vi "HIS_to_DAT_to_TRABS.vi"() -> ()   [LabVIEW 2015]
uses:
  DATA/HIS/HIS.lvclass
  dependecies/HIS_to_DAT_to_TRABS/cluster_template.ctl
panel:
  in  "file name TRABS":string
  in  "file name modifier DAT":string
  out "CERENKOV_unsel":T1(graph)
  out "BRUIT_unsel":T1(graph)
  out "BASE_sel":T1(graph)
  out "ABS_unsel":T1(graph)
  in  "select":bool caption="Lock"
  in  "Save TRABS":bool
  in  "Play":bool
  in  "Fast Forward":bool
  in  "Fast Reverse":bool
  in  "Skip to End":bool
  in  "Skip to Beginning":bool
  out "#CERENKOV":i32
  out "#BRUIT":i32
  out "#BASE":i32
  out "#ABS":i32
  in  "MAIN_path":path
  out "error out":errorcluster
  in  "to TRABS":bool
  out "TRABS":dbl[][](graph)
  in  "CERENKOV_b":bool
  in  "BRUIT_b":bool
  in  "BASE_b":bool
  out "CERENKOV_path":path
  out "BRUIT_path":path
  in  "stop_vi":bool
  in  "ABS_b":bool
  in  "All":bool
  in  "deselect":bool=TRUE caption="Lock"
  in  "Save DAT":bool
  out "BASE_path":path
  out "ABS_path":path
  out "CERENKOV DAT":dbl[][](graph)
  out "BRUIT DAT":dbl[][](graph)
  out "BASE DAT":dbl[][](graph)
  out "ABS DAT":dbl[][](graph)
  out "CERENKOV HIS":dbl[][](graph)
  out "BRUIT HIS":dbl[][](graph)
  out "BASE HIS":dbl[][](graph)
  in  "to Dat":bool
  out "ABS HIS":dbl[][](graph)
  out "Slide":u8(slide) scale=0.0..100.0
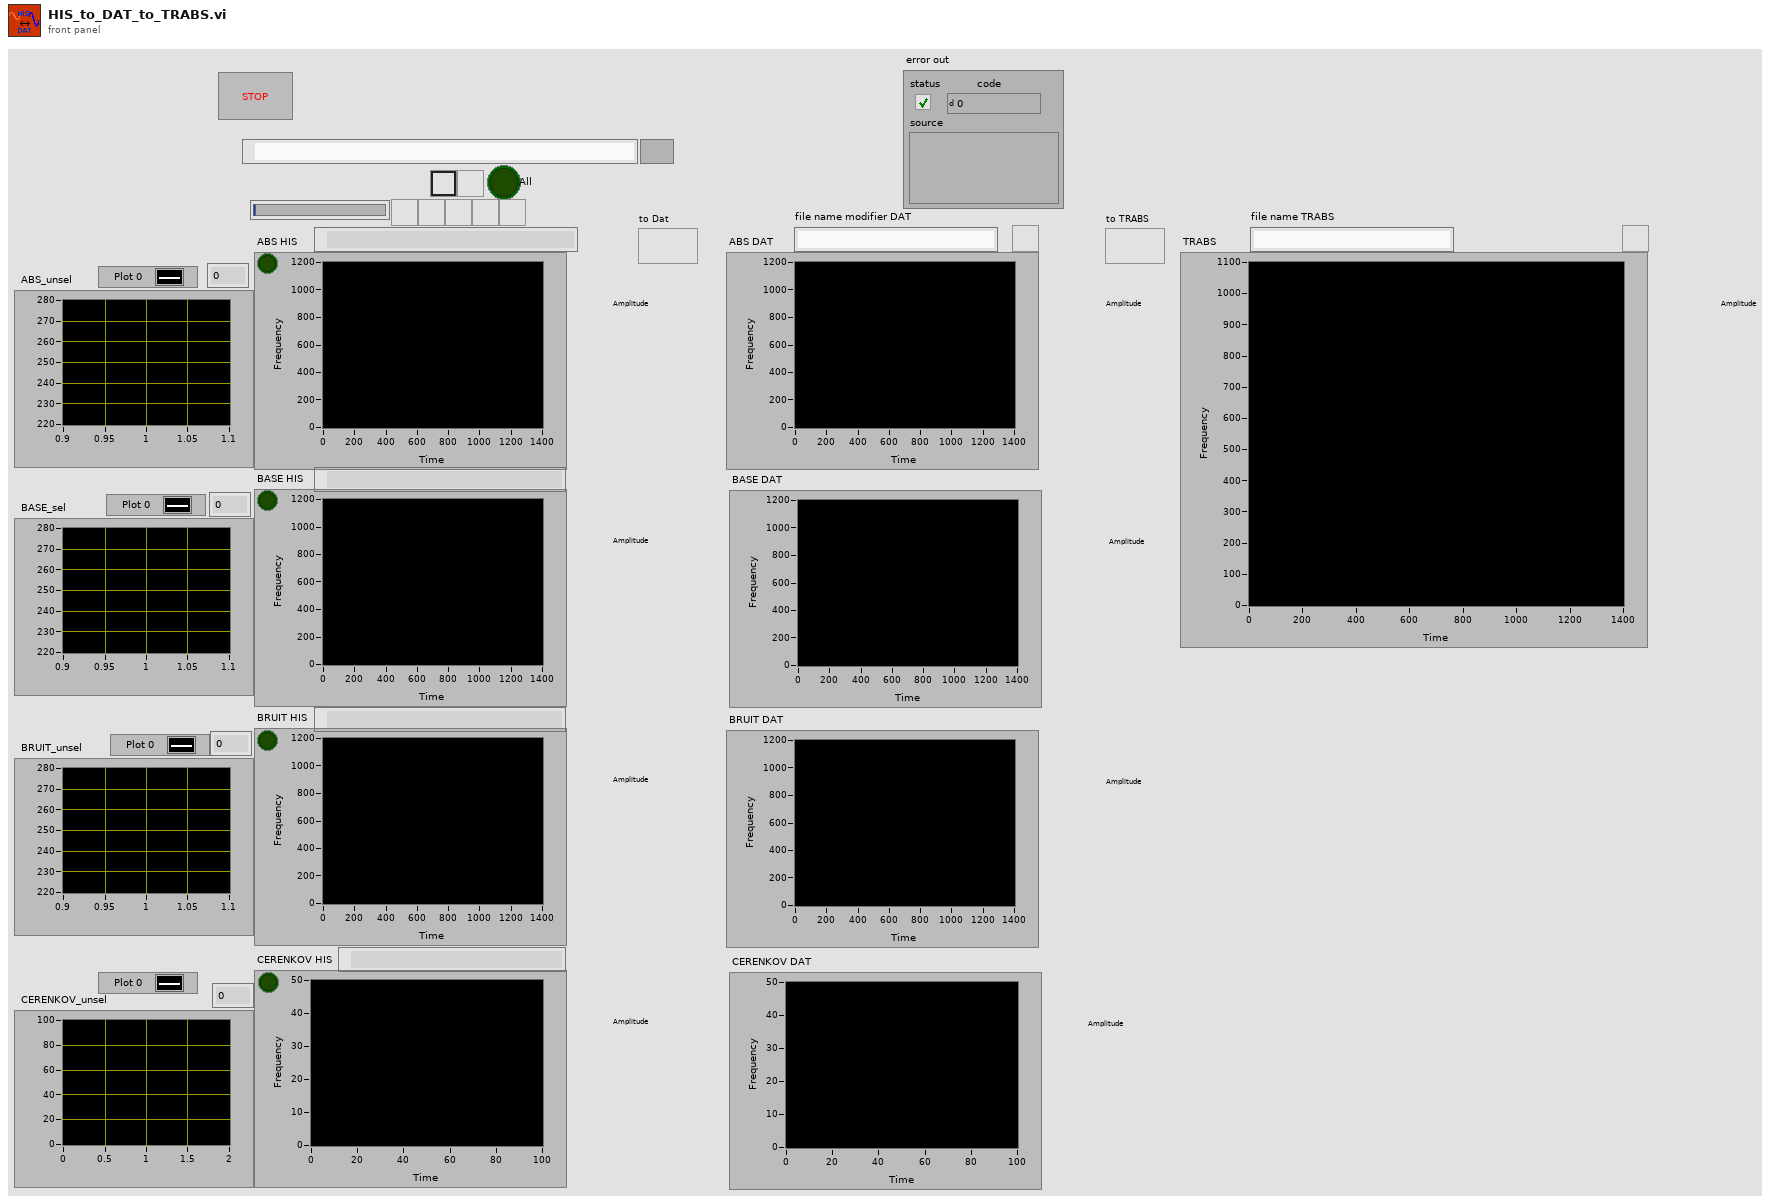
[diagram p1: front panel]
types:
  T1 = cluster{"appended array":dbl[], "appended array":dbl[]}
  T2 = typedef "cluster_template.ctl" = cluster{"HIS.lvclass":refnum<class "HIS.lvclass">, "selector":refnum<vi>, "HIS graph":refnum<vi>, "DAT graph":refnum<vi>, "path":refnum<vi>, "path MAIN":refnum<vi>, "#":refnum<vi>, "unsel Graph":refnum<vi>, "DATgraph":refnum<vi>}
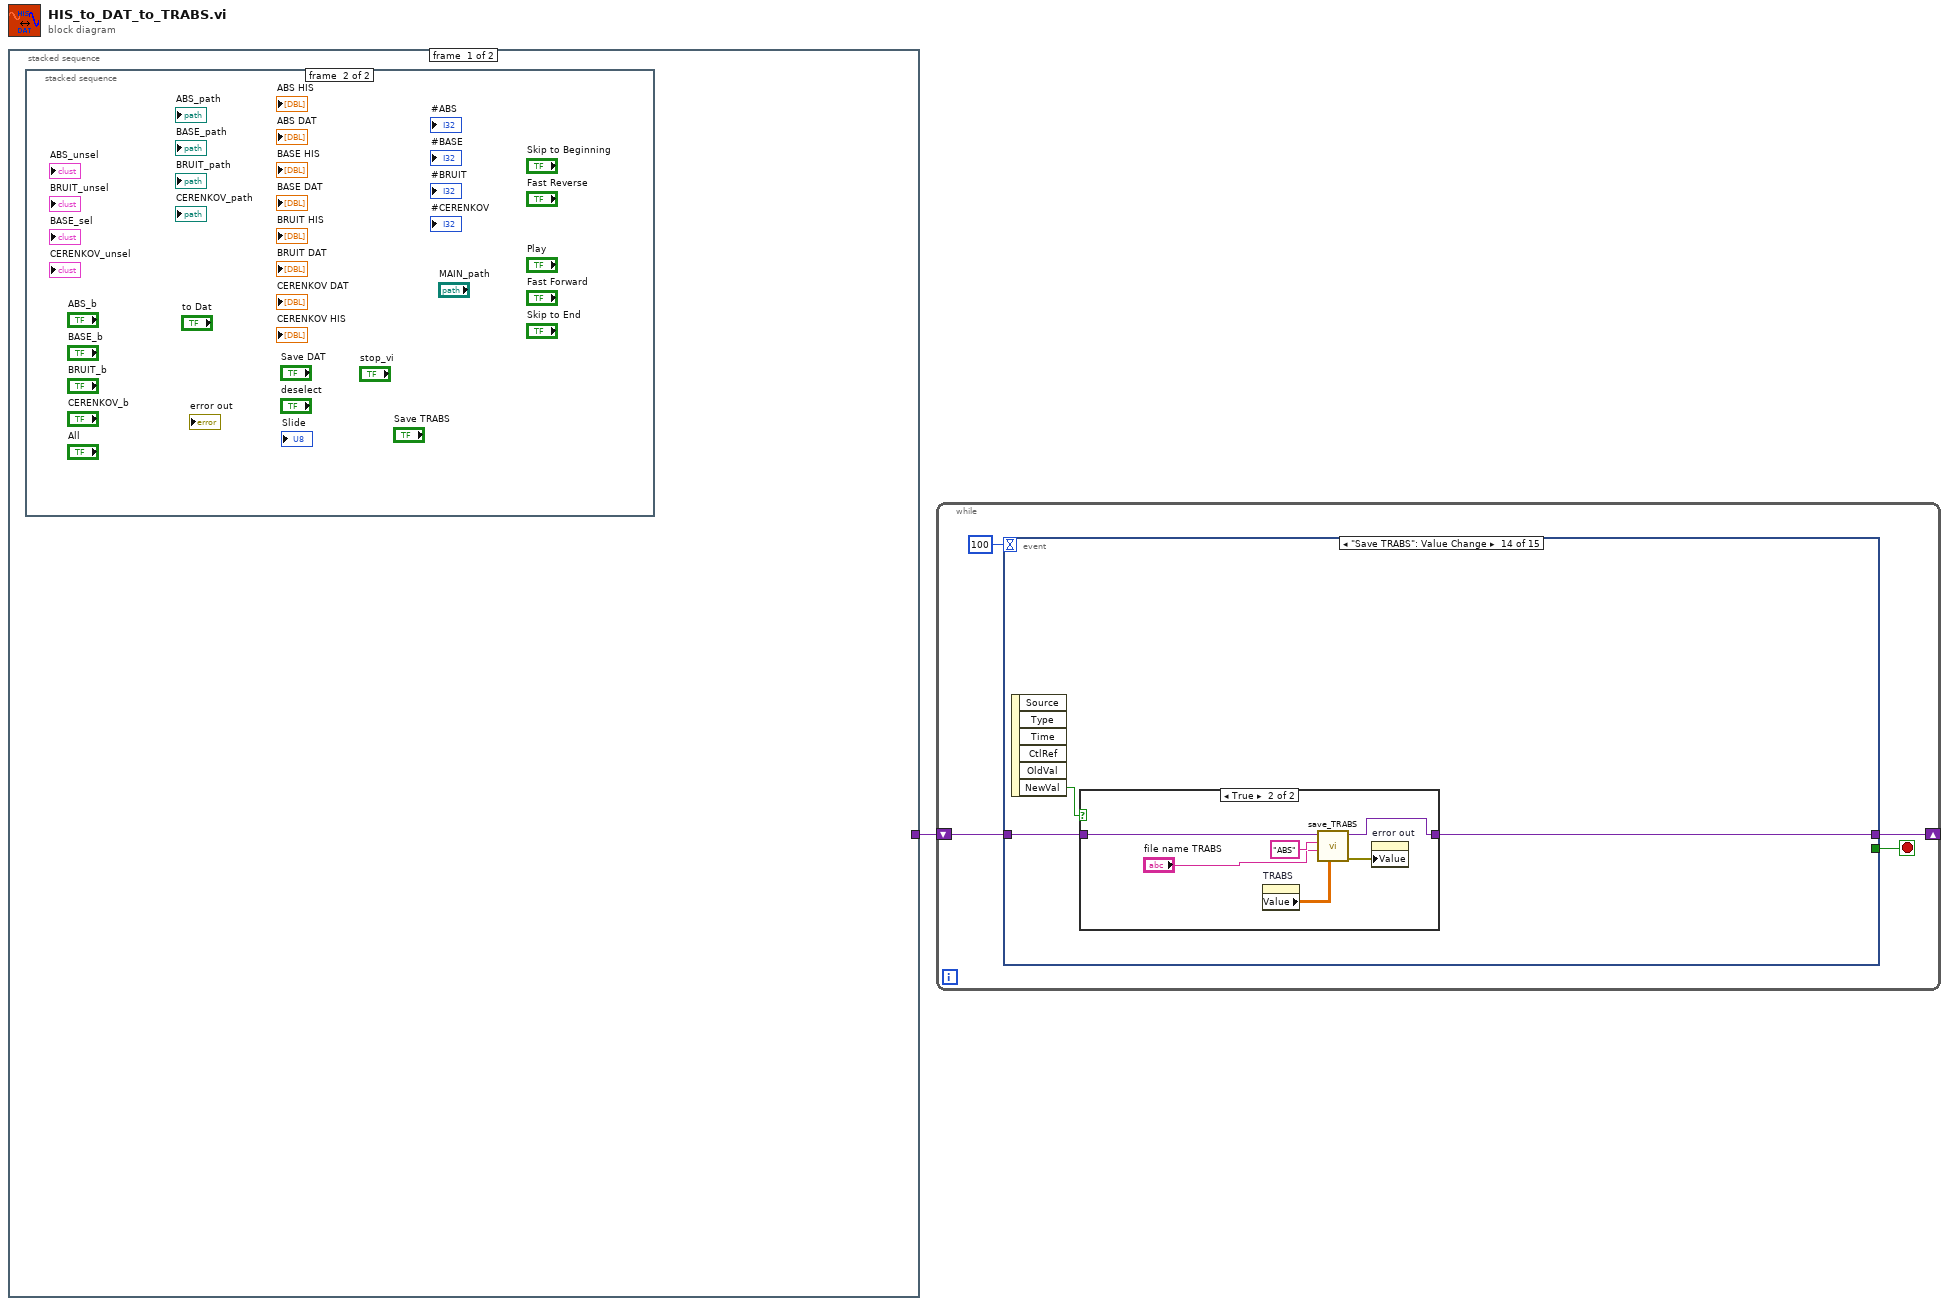
[diagram p0: block diagram]
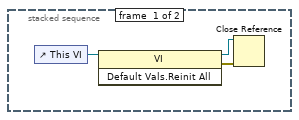
[diagram p2: hidden frame]
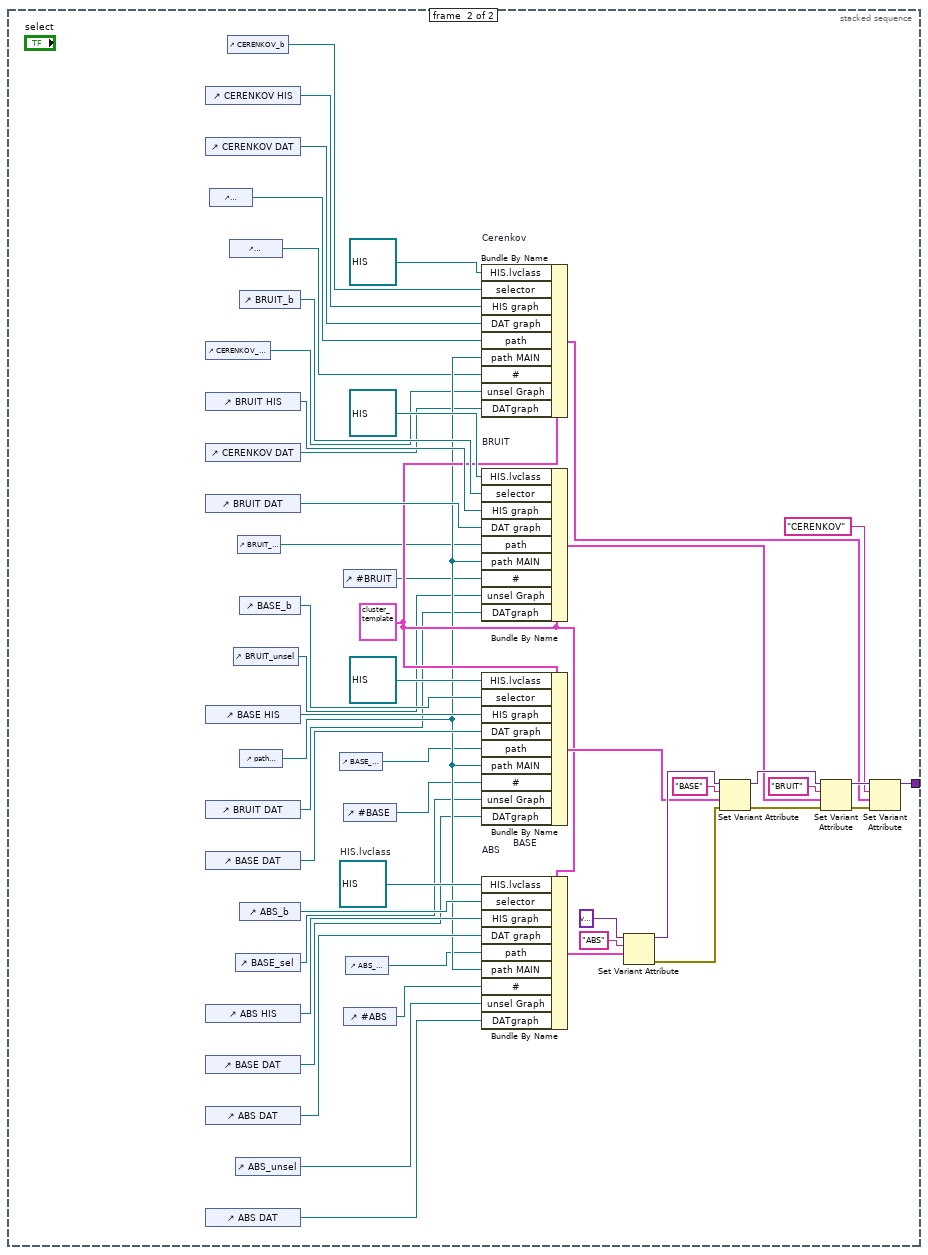
[diagram p3: hidden frame]
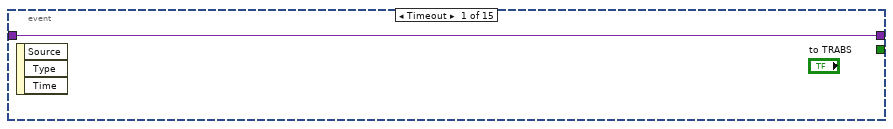
[diagram p4: hidden frame]
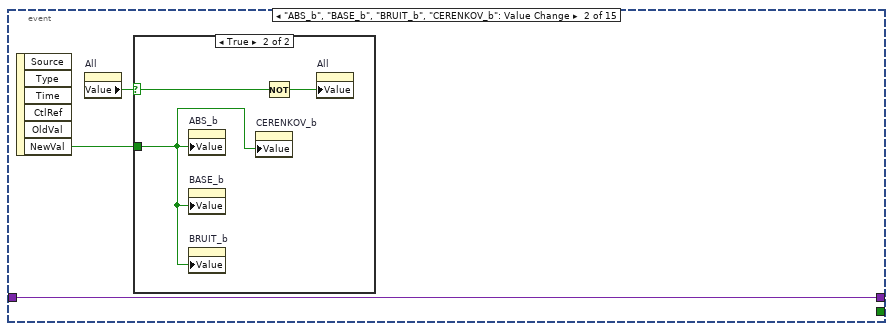
[diagram p5: hidden frame]
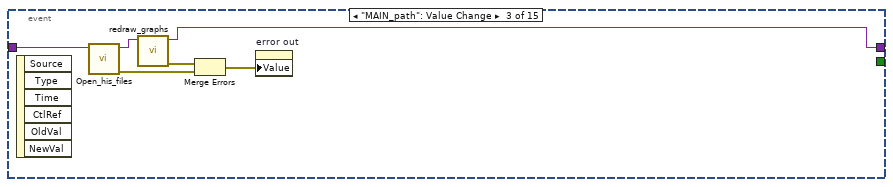
[diagram p7: hidden frame]
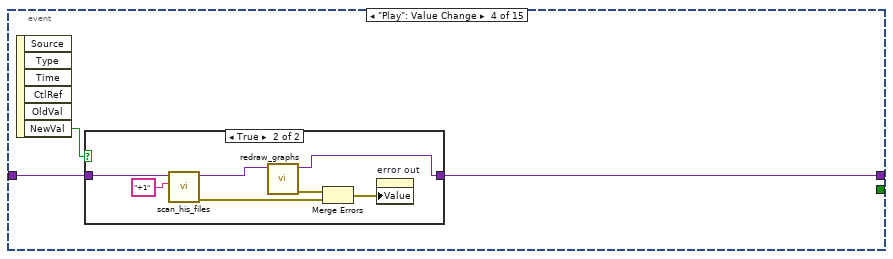
[diagram p8: hidden frame]
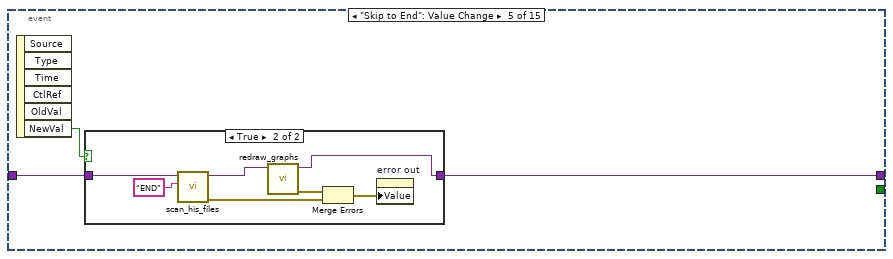
[diagram p10: hidden frame]
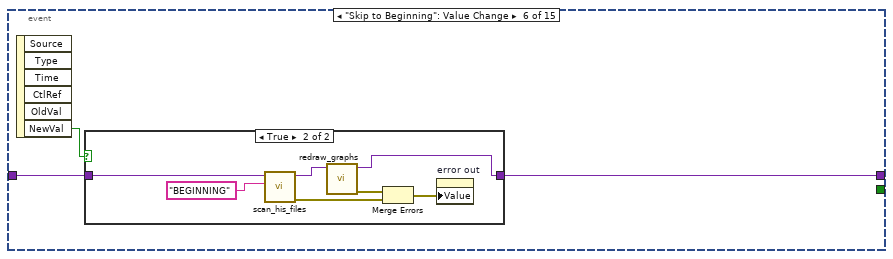
[diagram p12: hidden frame]
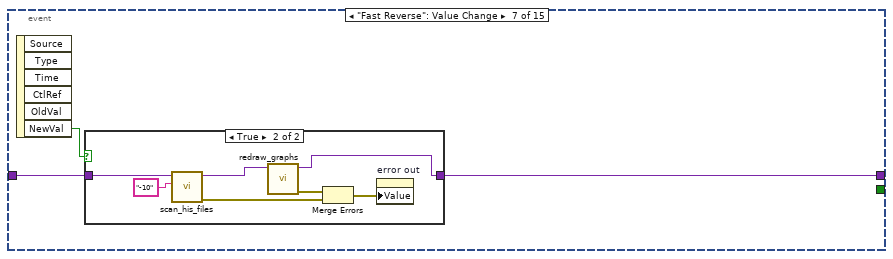
[diagram p14: hidden frame]
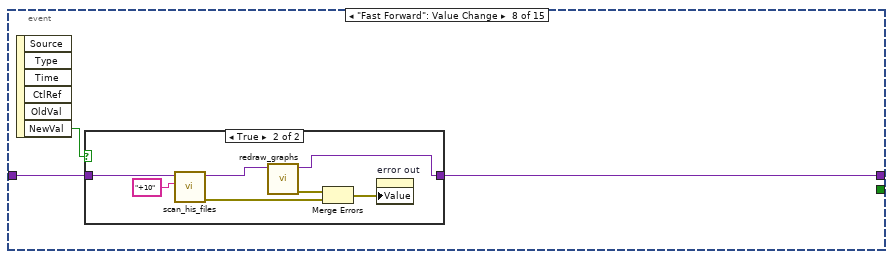
[diagram p16: hidden frame]
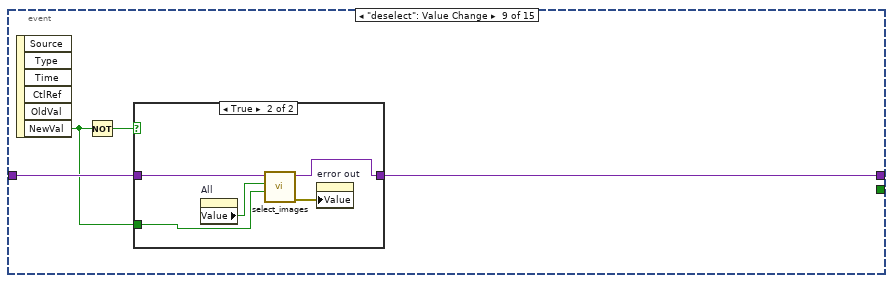
[diagram p18: hidden frame]
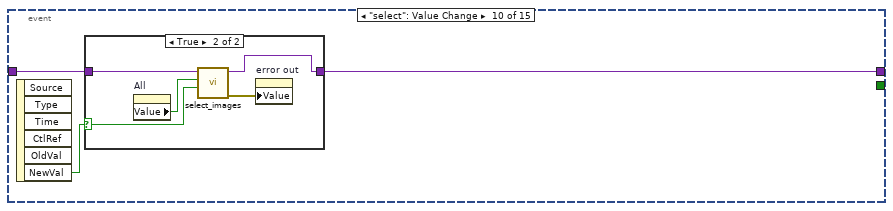
[diagram p20: hidden frame]
diagram:
  n1 = stacked-sequence {
    tunnel: [_ w44] -> w1
    frame #0 {
      n2 = stacked-sequence {
        frame #0 {
          n3 = control-ref of="This VI"() -> (w4:refnum<vi>)
          n4 = invoke class="VI" method="Default Vals.Reinit All"(reference=w4) -> (reference out=w3:refnum<vi>, error out=w2:errorcluster)  [unwired: 2 in, 1 out]
          n5 = Close Reference(reference=w3, error in (no error)=w2) -> ()  [unwired: 1 out]
        }
        frame #1 {
        }
      }
    }
    frame #1 {
      w28 = T2 {"HIS.lvclass"=refnum, "selector"=refnum, "HIS graph"=refnum, "DAT graph"=refnum, "path"=refnum, "path MAIN"=refnum, "#"=refnum, "unsel Graph"=refnum, "DATgraph"=refnum} ("output cluster")
      w42 = refnum<class "HIS.lvclass"> refnum  # HIS.lvclass
      n6 = control-ref of="CERENKOV HIS"() -> (w25:refnum<vi>)
      n7 = control-ref of="CERENKOV DAT"() -> (w26:refnum<vi>)
      n8 = control-ref of="CERENKOV_unsel"() -> (w11:refnum<vi>)
      n9 = control-ref of="BRUIT HIS"() -> (w31:refnum<vi>)
      n10 = control-ref of="CERENKOV DAT"() -> (w8:refnum<vi>)
      n11 = control-ref of="BRUIT DAT"() -> (w32:refnum<vi>)
      n12 = control-ref of="BASE HIS"() -> (w37:refnum<vi>)
      n13 = control-ref of="BRUIT DAT"() -> (w7:refnum<vi>)
      n14 = control-ref of="BASE DAT"() -> (w36:refnum<vi>)
      n15 = control-ref of="ABS HIS"() -> (w40:refnum<vi>)
      n16 = control-ref of="BASE DAT"() -> (w6:refnum<vi>)
      n17 = control-ref of="ABS DAT"() -> (w39:refnum<vi>)
      n18 = control-ref of="ABS DAT"() -> (w5:refnum<vi>)
      n19 = control-ref of="CERENKOV_path"() -> (w17:refnum<vi>)
      n20 = control-ref of="CERENKOV_b"() -> (w24:refnum<vi>)
      n21 = control-ref of="#CERENKOV"() -> (w15:refnum<vi>)
      n22 = control-ref of="BRUIT_unsel"() -> (w10:refnum<vi>)
      n23 = control-ref of="BASE_sel"() -> (w9:refnum<vi>)
      n24 = control-ref of="ABS_unsel"() -> (w12:refnum<vi>)
      n25 = control-ref of="BRUIT_path"() -> (w18:refnum<vi>)
      n26 = control-ref of="BRUIT_b"() -> (w33:refnum<vi>)
      n27 = control-ref of="BASE_b"() -> (w22:refnum<vi>)
      n28 = control-ref of="path MAIN"() -> (w21:refnum<vi>)
      n29 = control-ref of="ABS_b"() -> (w41:refnum<vi>)
      n30 = control-ref of="BASE_path"() -> (w20:refnum<vi>)
      n31 = control-ref of="#BRUIT"() -> (w13:refnum<vi>)
      n32 = control-ref of="#BASE"() -> (w16:refnum<vi>)
      n33 = control-ref of="#ABS"() -> (w14:refnum<vi>)
      n34 = control-ref of="ABS_path"() -> (w19:refnum<vi>)
      n35 = Bundle By Name "Cerenkov"(cluster=w28, "HIS.lvclass"=refnum<class "HIS.lvclass"> refnum, "selector"=w24, "HIS graph"=w25, "DAT graph"=w26, "path"=w17, "path MAIN"=w21, "#"=w15, "unsel Graph"=w11, "DATgraph"=w8) -> (w23:T2)
      n36 = Bundle By Name "BRUIT"(cluster=w28, "HIS.lvclass"=refnum<class "HIS.lvclass"> refnum, "selector"=w33, "HIS graph"=w31, "DAT graph"=w32, "path"=w18, "path MAIN"=w21, "#"=w13, "unsel Graph"=w10, "DATgraph"=w7) -> (w29:T2)
      n37 = Bundle By Name "BASE"(cluster=w28, "HIS.lvclass"=refnum<class "HIS.lvclass"> refnum, "selector"=w22, "HIS graph"=w37, "DAT graph"=w36, "path"=w20, "path MAIN"=w21, "#"=w16, "unsel Graph"=w9, "DATgraph"=w6) -> (w30:T2)
      n38 = Bundle By Name "ABS"(cluster=w28, "HIS.lvclass"=w42, "selector"=w41, "HIS graph"=w40, "DAT graph"=w39, "path"=w19, "path MAIN"=w21, "#"=w14, "unsel Graph"=w12, "DATgraph"=w5) -> (w38:T2)
      n39 = Set Variant Attribute(Variant=variant ("variant"), name="ABS", value=w38) -> (Variant out=w51:variant, error out=w53:errorcluster)  [unwired: 1 in, 1 out]
      n40 = Set Variant Attribute(Variant=w51, name="BASE", value=w30, error in=w53) -> (Variant out=w50:variant, error out=w46:errorcluster)  [unwired: 1 out]
      n41 = Set Variant Attribute(Variant=w50, name="BRUIT", value=w29, error in=w46) -> (Variant out=w48:variant, error out=w47:errorcluster)  [unwired: 1 out]
      n42 = Set Variant Attribute(Variant=w48, name="CERENKOV", value=w23, error in=w47) -> (Variant out=w44:variant)  [unwired: 2 out]
    }
  }
  n43 = while {
    shift-right: [w56] -> _
    shift-left: w1 -> [w55]
    stop <- w57 stop-if-true
    n44 = event shown="[13] \"Save TRABS\": Value Change" {
      selector: _ -> [_ _ _ _ _ _ _ _ _ _ _ _ _ _ _]
      dyn-events: _ -> [_ _ _ _ _ _ _ _ _ _ _ _ _ _ _]
      timeout: 100 -> [_ _ _ _ _ _ _ _ _ _ _ _ _ _ _]
      tunnel: [_ _ _ _ _ _ _ _ _ _ _ _ _ _ w201] -> w57
      tunnel: [w59 w62 w70 w73 w84 w95 w106 w117 w129 w138 w146 w153 w162 w190 w200] -> w56
      tunnel: w55 -> [w59 w62 w69 w74 w85 w96 w107 w118 w130 w139 w148 w155 w162 w192 w200]
      event Timeout {
        n45 = event-data() -> ()  [unwired: 1 in, 3 out]
      }
      event "ABS_b", "BASE_b", "BRUIT_b", "CERENKOV_b": Value Change {
        n46 = event-data() -> ("NewVal"=w60:bool)  [unwired: 1 in, 5 out]
        n47 = property on="All" class="Bool (strict)"() -> ("Value"=w61:bool)  [unwired: 2 in, 2 out]
        n48 = case shown="True" w61 {
          selector: w61 -> [_ w65]
          tunnel: w60 -> [_ w63]
          frame False {
          }
          frame True {
            n49 = property on="ABS_b" class="Bool (strict)"("Value"=w63) -> ()  [unwired: 2 in, 2 out]
            n50 = property on="BASE_b" class="Bool (strict)"("Value"=w63) -> ()  [unwired: 2 in, 2 out]
            n51 = property on="BRUIT_b" class="Bool (strict)"("Value"=w63) -> ()  [unwired: 2 in, 2 out]
            n52 = property on="CERENKOV_b" class="Bool (strict)"("Value"=w63) -> ()  [unwired: 2 in, 2 out]
            n53 = Not(x=w65) -> (.not. x?=w64:bool)
            n54 = property on="All" class="Bool (strict)"("Value"=w64) -> ()  [unwired: 2 in, 2 out]
          }
        }
      }
      event "MAIN_path": Value Change {
        n55 = event-data() -> ()  [unwired: 1 in, 6 out]
        n56 = call "Open_his_files.vi"("dict of HIS IN"=w69) -> ("error out"=w67:errorcluster, "dict of HIS OUT"=w71:variant)  [unwired: 9 in]
        n57 = call "redraw_graphs.vi"("dict of HIS IN"=w71) -> ("error out"=w68:errorcluster, "dict of HIS OUT"=w70:variant)  [unwired: 9 in]
        n58 = Merge Errors(w68, w67) -> (w66:errorcluster)
        n59 = property on="error out" class="Clust (strict)"("Value"=w66) -> ()  [unwired: 2 in, 2 out]
      }
      event "Play": Value Change {
        n60 = event-data() -> ("NewVal"=w72:bool)  [unwired: 1 in, 5 out]
        n61 = case shown="True" w72 {
          tunnel: w74 -> [w75 w82]
          tunnel: [w75 w80] -> w73
          frame False {
          }
          frame True {
            n62 = call "scan_his_files.vi"("Control"="+1", "dict of HIS IN"=w82) -> ("error out"=w77:errorcluster, "dict of HIS OUT"=w81:variant)  [unwired: 8 in]
            n63 = call "redraw_graphs.vi"("dict of HIS IN"=w81) -> ("error out"=w78:errorcluster, "dict of HIS OUT"=w80:variant)  [unwired: 9 in]
            n64 = Merge Errors(w78, w77) -> (w79:errorcluster)
            n65 = property on="error out" class="Clust (strict)"("Value"=w79) -> ()  [unwired: 2 in, 2 out]
          }
        }
      }
      event "Skip to End": Value Change {
        n66 = event-data() -> ("NewVal"=w83:bool)  [unwired: 1 in, 5 out]
        n67 = case shown="True" w83 {
          tunnel: w85 -> [w86 w93]
          tunnel: [w86 w91] -> w84
          frame False {
          }
          frame True {
            n68 = call "scan_his_files.vi"("Control"="END", "dict of HIS IN"=w93) -> ("error out"=w88:errorcluster, "dict of HIS OUT"=w92:variant)  [unwired: 8 in]
            n69 = call "redraw_graphs.vi"("dict of HIS IN"=w92) -> ("error out"=w89:errorcluster, "dict of HIS OUT"=w91:variant)  [unwired: 9 in]
            n70 = Merge Errors(w89, w88) -> (w90:errorcluster)
            n71 = property on="error out" class="Clust (strict)"("Value"=w90) -> ()  [unwired: 2 in, 2 out]
          }
        }
      }
      event "Skip to Beginning": Value Change {
        n72 = event-data() -> ("NewVal"=w94:bool)  [unwired: 1 in, 5 out]
        n73 = case shown="True" w94 {
          tunnel: w96 -> [w97 w104]
          tunnel: [w97 w102] -> w95
          frame False {
          }
          frame True {
            n74 = call "scan_his_files.vi"("Control"="BEGINNING", "dict of HIS IN"=w104) -> ("error out"=w99:errorcluster, "dict of HIS OUT"=w103:variant)  [unwired: 8 in]
            n75 = call "redraw_graphs.vi"("dict of HIS IN"=w103) -> ("error out"=w100:errorcluster, "dict of HIS OUT"=w102:variant)  [unwired: 9 in]
            n76 = Merge Errors(w100, w99) -> (w101:errorcluster)
            n77 = property on="error out" class="Clust (strict)"("Value"=w101) -> ()  [unwired: 2 in, 2 out]
          }
        }
      }
      event "Fast Reverse": Value Change {
        n78 = event-data() -> ("NewVal"=w105:bool)  [unwired: 1 in, 5 out]
        n79 = case shown="True" w105 {
          tunnel: w107 -> [w108 w115]
          tunnel: [w108 w113] -> w106
          frame False {
          }
          frame True {
            n80 = call "scan_his_files.vi"("Control"="-10", "dict of HIS IN"=w115) -> ("error out"=w110:errorcluster, "dict of HIS OUT"=w114:variant)  [unwired: 8 in]
            n81 = call "redraw_graphs.vi"("dict of HIS IN"=w114) -> ("error out"=w111:errorcluster, "dict of HIS OUT"=w113:variant)  [unwired: 9 in]
            n82 = Merge Errors(w111, w110) -> (w112:errorcluster)
            n83 = property on="error out" class="Clust (strict)"("Value"=w112) -> ()  [unwired: 2 in, 2 out]
          }
        }
      }
      event "Fast Forward": Value Change {
        n84 = event-data() -> ("NewVal"=w116:bool)  [unwired: 1 in, 5 out]
        n85 = case shown="True" w116 {
          tunnel: w118 -> [w119 w126]
          tunnel: [w119 w124] -> w117
          frame False {
          }
          frame True {
            n86 = call "scan_his_files.vi"("Control"="+10", "dict of HIS IN"=w126) -> ("error out"=w121:errorcluster, "dict of HIS OUT"=w125:variant)  [unwired: 8 in]
            n87 = call "redraw_graphs.vi"("dict of HIS IN"=w125) -> ("error out"=w122:errorcluster, "dict of HIS OUT"=w124:variant)  [unwired: 9 in]
            n88 = Merge Errors(w122, w121) -> (w123:errorcluster)
            n89 = property on="error out" class="Clust (strict)"("Value"=w123) -> ()  [unwired: 2 in, 2 out]
          }
        }
      }
      event "deselect": Value Change {
        n90 = event-data() -> ("NewVal"=w127:bool)  [unwired: 1 in, 5 out]
        n91 = Not(x=w127) -> (.not. x?=w128:bool)
        n92 = case shown="True" w128 {
          tunnel: w130 -> [w131 w136]
          tunnel: [w131 w135] -> w129
          tunnel: w127 -> [_ w133]
          frame False {
          }
          frame True {
            n93 = property on="All" class="Bool (strict)"() -> ("Value"=w132:bool)  [unwired: 2 in, 2 out]
            n94 = call "select_images.vi"("Select"=w133, "All"=w132, "dict of HIS IN"=w136) -> ("error out"=w134:errorcluster, "dict of HIS OUT"=w135:variant)  [unwired: 7 in]
            n95 = property on="error out" class="Clust (strict)"("Value"=w134) -> ()  [unwired: 2 in, 2 out]
          }
        }
      }
      event "select": Value Change {
        n96 = event-data() -> ("NewVal"=w137:bool)  [unwired: 1 in, 5 out]
        n97 = case shown="True" w137 {
          selector: w137 -> [_ w141]
          tunnel: w139 -> [w140 w145]
          tunnel: [w140 w144] -> w138
          frame False {
          }
          frame True {
            n98 = property on="All" class="Bool (strict)"() -> ("Value"=w142:bool)  [unwired: 2 in, 2 out]
            n99 = call "select_images.vi"("Select"=w141, "All"=w142, "dict of HIS IN"=w145) -> ("error out"=w143:errorcluster, "dict of HIS OUT"=w144:variant)  [unwired: 7 in]
            n100 = property on="error out" class="Clust (strict)"("Value"=w143) -> ()  [unwired: 2 in, 2 out]
          }
        }
      }
      event "to Dat": Value Change {
        n101 = event-data() -> ("NewVal"=w147:bool)  [unwired: 1 in, 5 out]
        n102 = case shown="True" w147 {
          tunnel: w148 -> [w149 w152]
          tunnel: [w149 w151] -> w146
          frame False {
          }
          frame True {
            n103 = call "update_DAT_graphs.vi"("dict of HIS IN"=w152) -> ("error out"=w150:errorcluster, "dict of HIS OUT"=w151:variant)  [unwired: 9 in]
            n104 = property on="error out" class="Clust (strict)"("Value"=w150) -> ()  [unwired: 2 in, 2 out]
          }
        }
      }
      event "Save DAT": Value Change {
        n105 = event-data() -> ("NewVal"=w154:bool)  [unwired: 1 in, 5 out]
        n106 = case shown="True" w154 {
          tunnel: w155 -> [w156 w160]
          tunnel: [w156 w159] -> w153
          frame False {
          }
          frame True {
            n107 = call "save_dat.vi"("modifier"="file name modifier DAT", "dict of HIS IN"=w160) -> ("error out"=w158:errorcluster, "dict of HIS OUT"=w159:variant)  [unwired: 8 in]
            n108 = property on="error out" class="Clust (strict)"("Value"=w158) -> ()  [unwired: 2 in, 2 out]
          }
        }
      }
      event "to TRABS": Value Change {
        n109 = event-data() -> ("NewVal"=w161:bool)  [unwired: 1 in, 5 out]
        n110 = case shown="True" w161 {
          frame False {
          }
          frame True {
            n111 = property on="CERENKOV DAT" class="IntGraph (strict)"() -> ("Value"=w173:dbl[][])  [unwired: 2 in, 2 out]
            n112 = property on="BRUIT DAT" class="IntGraph (strict)"() -> ("Value"=w171:dbl[][])  [unwired: 2 in, 2 out]
            n113 = property on="ABS DAT" class="IntGraph (strict)"() -> ("Value"=w170:dbl[][])  [unwired: 2 in, 2 out]
            n114 = Empty Array?(array=w171) -> (empty?=w172:bool)
            n115 = Empty Array?(array=w173) -> (empty?=w174:bool)
            n116 = case shown="True" w172 {
              tunnel: w170 -> [_ w182]
              tunnel: [w176 w177] -> w169
              tunnel: w171 -> [w176 _]
              frame False {
              }
              frame True {
                n117 = Array Size(array=w182) -> (size(s)=w181:i32[])
                n118 = Index Array(array=w181) -> (element #1=w179:i32, element #2=w178:i32)  [unwired: 2 in]
                n119 = Initialize Array(0.0 ("element"), w179, w178) -> (w177:dbl[][])
              }
            }
            n120 = case shown="False" w174 {
              tunnel: w170 -> [_ w189]
              tunnel: [w183 w184] -> w167
              tunnel: w173 -> [w183 _]
              frame False {
              }
              frame True {
                n121 = Array Size(array=w189) -> (size(s)=w188:i32[])
                n122 = Index Array(array=w188) -> (element #1=w186:i32, element #2=w185:i32)  [unwired: 2 in]
                n123 = Initialize Array(0.0 ("element"), w186, w185) -> (w184:dbl[][])
              }
            }
            n124 = property on="BASE DAT" class="IntGraph (strict)"() -> ("Value"=w175:dbl[][])  [unwired: 2 in, 2 out]
            n125 = Subtract(x=w170, y=w169) -> (x-y=w168:dbl[][])
            n126 = Subtract(x=w175, y=w169) -> (x-y=w166:dbl[][])
            n127 = Subtract(x=w168, y=w167) -> (x-y=w165:dbl[][])
            n128 = Divide(x=w166, y=w165) -> (x/y=w164:dbl[][])
            n129 = Logarithm Base 10(1:w164) -> (0:→"TRABS":dbl[][])
          }
        }
      }
      event "Save TRABS": Value Change {
        n130 = event-data() -> ("NewVal"=w191:bool)  [unwired: 1 in, 5 out]
        n131 = case shown="True" w191 {
          tunnel: w192 -> [w193 w199]
          tunnel: [w193 w197] -> w190
          frame False {
          }
          frame True {
            n132 = property on="TRABS" class="IntGraph (strict)"() -> ("Value"=w195:dbl[][])  [unwired: 2 in, 2 out]
            n133 = call "save_TRABS.vi"("TRABS"=w195, "filename"="file name TRABS", "type"="ABS", "dict of HIS IN"=w199) -> ("error out"=w194:errorcluster, "dict of HIS OUT"=w197:variant)  [unwired: 6 in]
            n134 = property on="error out" class="Clust (strict)"("Value"=w194) -> ()  [unwired: 2 in, 2 out]
          }
        }
      }
      event "stop_vi": Value Change {
        n135 = event-data() -> ("NewVal"=w201:bool)  [unwired: 1 in, 5 out]
      }
    }
  }
